vi "CalculateChargeDensity.vi"(6 "empty image":bool, 8 "Final":T2, 9 "Settings.LimitE":T1, 10 "MaxE":dbl, 11 "Z":dbl[][](graph)) -> (0 "Charge vs angle":cluster{"Ramp Pattern":dbl[], dbl[]}, 1 "Integrated spectrum (attoC/MeV or GeV?)":cluster{"Momentum [MeV/C]":dbl[], dbl[]}(graph), 2 "charge (sum)":dbl, 3 "charge density":dbl[][](array[numeric]), 5 "time: 2Dinter":u32)   [LabVIEW 2013]
uses:
  Controls/finalCalib--Cluster.ctl
  shared/OnOffTypeDef.ctl
  <vilib>/Analysis/8numeric.llb/1D Numeric Integration.vi
  <vilib>/gmath/interp.llb/Interpolate 2D (2d X,Y).vi
  <vilib>/Analysis/NI_AALPro.lvlib
  <vilib>/gmath/NI_Gmath.lvlib
panel:
  out "mask":dbl[][](graph)
  out "Out":dbl[][](array[numeric])
  out "xi":dbl[][](array[numeric])
  out "transposed array 2":dbl[][](graph)
  out "transposed array":dbl[][](graph)
  in  "error constant":errorcluster
  out "error":i32
  out "Intensity Graph":dbl[][](graph)
  out "time: spectra":u32
  out "charge (YSum)":dbl format="%0.4f"
  out "charge (spectra)":dbl format="%0.4f"
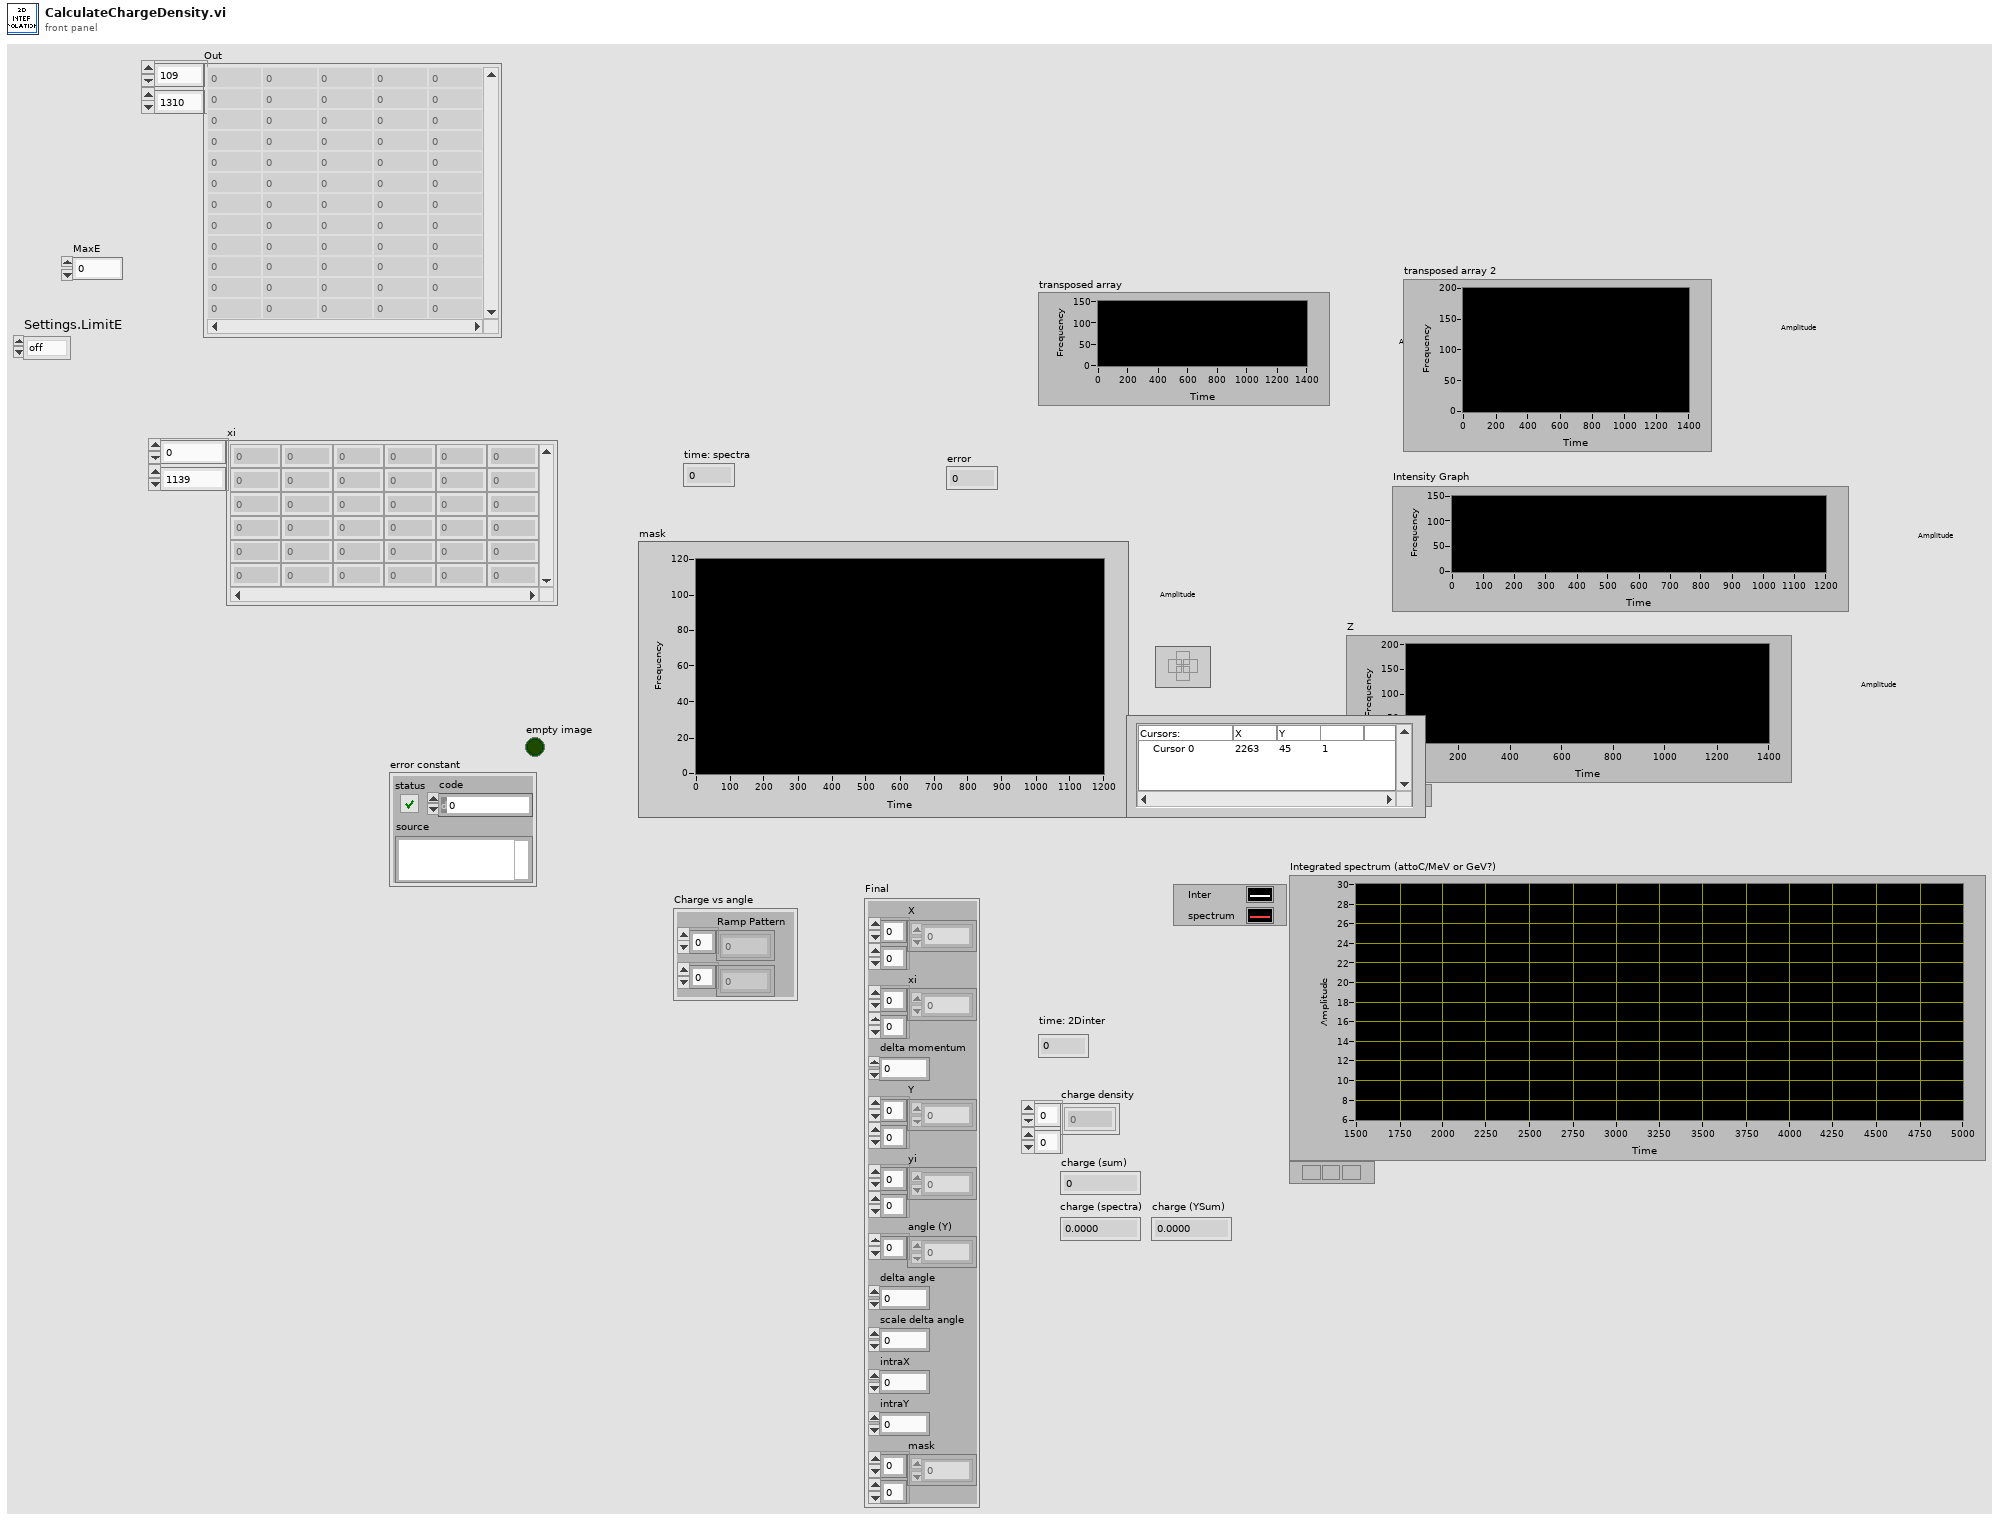
[diagram p1: front panel]
types:
  T1 = typedef "OnOffTypeDef.ctl" = enum16{"off", "on"}
  T2 = typedef "finalCalib--Cluster.ctl" = cluster{"X":dbl[][], "xi":dbl[][], "delta momentum":dbl, "Y":dbl[][], "yi":dbl[][], "angle (Y)":dbl[], "delta angle":dbl, "scale delta angle":dbl, "intraX":dbl, "intraY":dbl, "mask":dbl[][]}
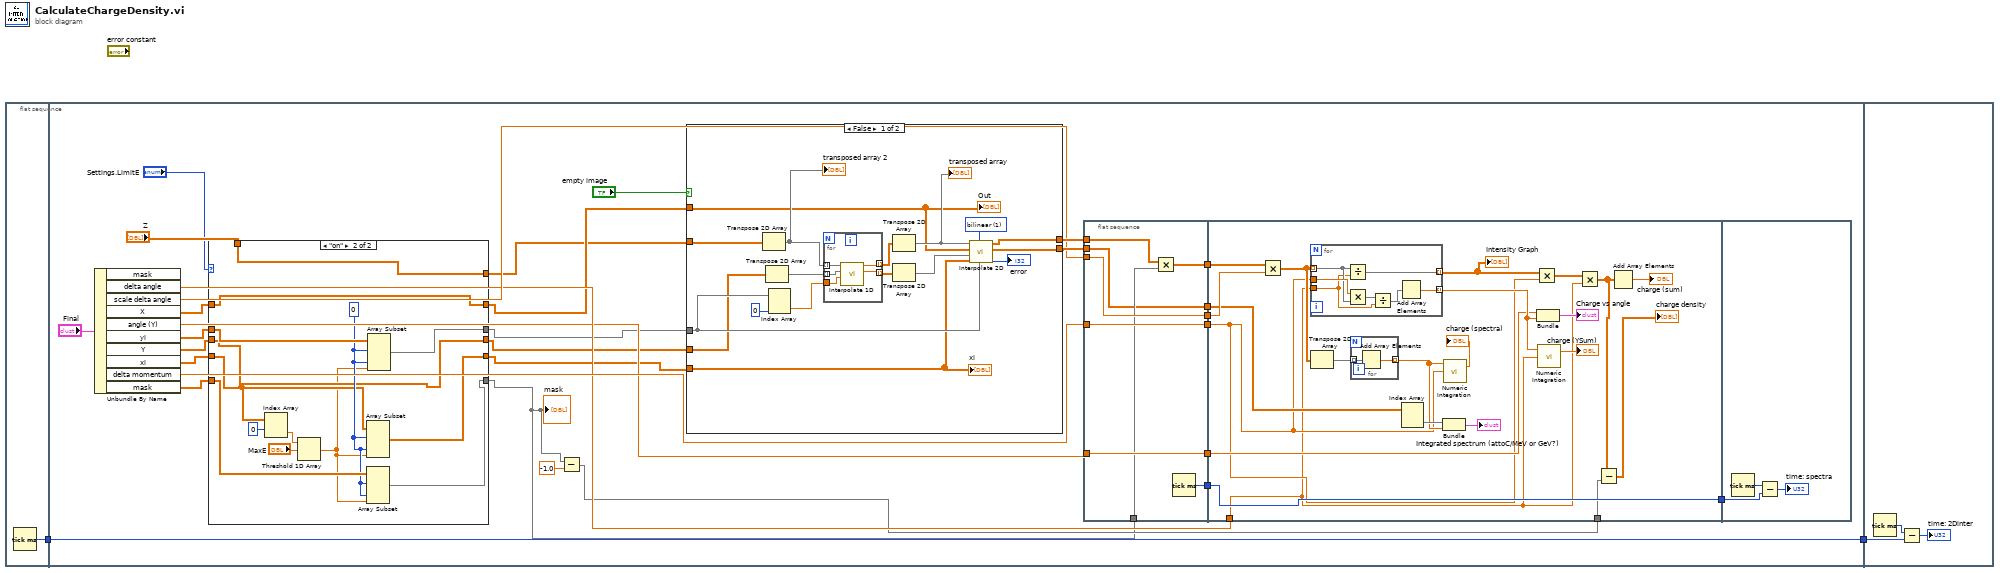
[diagram p0: block diagram]
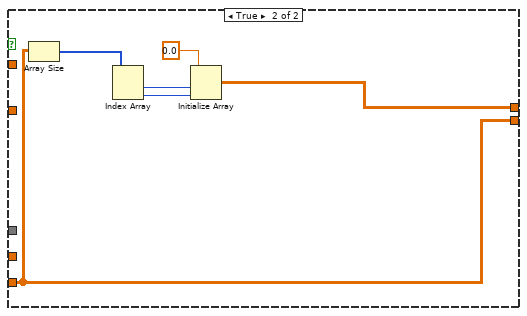
[diagram p3: hidden frame]
diagram:
  n1 = flat-sequence {
    tunnel: [w3] -> w2
    tunnel: w2 -> [w34]
    tunnel: [w34] -> w1
    tunnel: w1 -> [w126]
    frame #0 {
      n2 = Tick Count (ms)() -> (millisecond timer value=w3:u32)
    }
    frame #1 {
      n3 = Unbundle By Name("Final") -> ("delta angle"=w21:dbl, "scale delta angle"=w31:dbl, "X"=w16:dbl[][], "angle (Y)"=w20:dbl[], "yi"=w14:dbl[][], "Y"=w13:dbl[][], "xi"=w12:dbl[][], "delta momentum"=w23:dbl, "mask"=w8:dbl[][])  [unwired: 1 out]
      n4 = case shown="\"on\"" "Settings.LimitE" {
        tunnel: w16 -> [w40 w47]
        tunnel: [w40 w47] -> w15
        tunnel: w14 -> [w39 w54]
        tunnel: [w39 w53] -> w5
        tunnel: w13 -> [w38 w46]
        tunnel: [w38 w46] -> w6
        tunnel: w12 -> [w37 w45]
        tunnel: [w37 w52] -> w11
        tunnel: w8 -> [w36 w51]
        tunnel: [w36 w50] -> w7
        tunnel: "Z" -> [w35 w48]
        tunnel: [w35 w48] -> w9
        frame "off", Default {
        }
        frame "on" {
          w49 = 0 ("index")
          n5 = Index Array(array=w45, index (row)=0) -> (element=w43:dbl[])  [unwired: 1 in]
          n6 = Threshold 1D Array(2:"MaxE", 3:w43) -> (0:w41:dbl)  [unwired: 1 in]
          n7 = Array Subset(array=w45, index (row)=w49, index (col)=w49, length (col)=w41) -> (w52:dbl[][])  [unwired: 1 in]
          n8 = Array Subset(array=w51, index (row)=w49, index (col)=w49, length (col)=w41) -> (w50:dbl[][])  [unwired: 1 in]
          n9 = Array Subset(array=w54, index (row)=w49, index (col)=w49, length (col)=w41) -> (w53:dbl[][])  [unwired: 1 in]
        }
      }
      "mask" <- w7
      n10 = Subtract(x=w7, y=-1.0) -> (x-y=w17:dbl[][])
      n11 = case shown="False" "empty image" {
        tunnel: w15 -> [w56 _]
        tunnel: [w70 w81] -> w33
        tunnel: w11 -> [w57 w81]
        tunnel: w9 -> [w55 _]
        tunnel: [w71 w77] -> w32
        tunnel: w6 -> [w58 _]
        tunnel: w5 -> [w60 _]
        frame False {
          w66 = 1 items=["nearest", "bilinear", "bicubic", "bicubic spline"] ("method")
          n12 = Transpose 2D Array(2D array=w55) -> (transposed array=w59:dbl[][])
          "transposed array 2" <- w59
          n13 = Transpose 2D Array(2D array=w58) -> (transposed array=w68:dbl[][])
          n14 = Index Array(array=w60, index (col)=0 ("disabled index (col)")) -> (element=w67:dbl[])  [unwired: 1 in]
          n15 = for {
            tunnel: w59 -> [w76] mode=indexing
            tunnel: w68 -> [w75] mode=indexing
            tunnel: w67 -> [w74]
            tunnel: [w73] -> w64 mode=indexing
            tunnel: [w72] -> w63 mode=indexing
            n16 = call <vilib>:"Interpolate 1D.vi"("xi"=w74, "X"=w75, "Y"=w76) -> ("xi used"=w72:dbl[], "yi"=w73:dbl[])  [unwired: 6 in, 1 out]
          }
          n17 = Transpose 2D Array(2D array=w64) -> (transposed array=w62:dbl[][])
          "transposed array" <- w62
          n18 = Transpose 2D Array(2D array=w63) -> (transposed array=w61:dbl[][])
          n19 = call-poly <vilib>:"Interpolate 2D.vi"("yi"=w60, "method"=w66, "xi"=w57, "Y"=w61, "X"=w56, "Z"=w62) -> ("error"=→"error":i32, "xi used"=w70:dbl[][], "zi"=w71:dbl[][])  [unwired: 2 in, 1 out]
          "xi" <- w57
          "Out" <- w56
        }
        frame True {
          n20 = Array Size(array=w81) -> (size(s)=w80:i32[])
          n21 = Index Array(array=w80) -> (element #1=w79:i32, element #2=w78:i32)  [unwired: 2 in]
          n22 = Initialize Array(0.0 ("element"), w79, w78) -> (w77:dbl[][])
        }
      }
      n23 = flat-sequence {
        tunnel: w31 -> [w89]
        tunnel: w32 -> [w86]
        tunnel: w20 -> [w90]
        tunnel: w33 -> [w83]
        tunnel: [w83] -> w30
        tunnel: [w90] -> w29
        tunnel: [w84] -> w28
        tunnel: [w89] -> w27
        tunnel: [w88] -> w26
        tunnel: w23 -> [w87]
        tunnel: [w87] -> w22
        tunnel: w7 -> [w85]
        tunnel: w21 -> [w95]
        tunnel: w30 -> [w100]
        tunnel: w29 -> [w105]
        tunnel: w28 -> [w103]
        tunnel: w27 -> [w102]
        tunnel: w26 -> [w101]
        tunnel: [w101] -> w25
        tunnel: w22 -> [w97]
        tunnel: w17 -> [w92]
        tunnel: w25 -> [w123]
        frame #0 {
          n24 = Multiply(x=w86, y=w85) -> (x*y=w84:dbl[][])
          n25 = Tick Count (ms)() -> (millisecond timer value=w88:u32)
        }
        frame #1 {
          n26 = Multiply(x=w103, y=w102) -> (x*y=w99:dbl[][])
          n27 = for {
            tunnel: w99 -> [w117] mode=indexing
            tunnel: [w121] -> w106 mode=indexing
            tunnel: w97 -> [w118]
            tunnel: w95 -> [w116]
            tunnel: [w115] -> w98 mode=indexing
            n28 = Divide(x=w117, y=w116) -> (x/y=w115:dbl[])
            n29 = Multiply(x=w118, y=w117) -> (x*y=w120:dbl[])
            n30 = Divide(x=w120, y=w116) -> (x/y=w119:dbl[])
            n31 = Add Array Elements(numeric array=w119) -> (sum=w121:dbl)
          }
          "Intensity Graph" <- w98
          n32 = Transpose 2D Array(2D array=w99) -> (transposed array=w112:dbl[][])
          n33 = for {
            tunnel: w112 -> [w113] mode=indexing
            tunnel: [w114] -> w109 mode=indexing
            n34 = Add Array Elements(numeric array=w113) -> (sum=w114:dbl)
          }
          n35 = Index Array(array=w100) -> (element=w110:dbl[])  [unwired: 2 in]
          n36 = Bundle("xi"=w110, w109) -> (→"Integrated spectrum (attoC/MeV or GeV?)":cluster{"xi":dbl[], dbl[]})  [unwired: 1 in]
          n37 = call-poly <vilib>:"Numeric Integration.vi"("dt"=w97, "Input Array"=w109) -> ("result"=→"charge (spectra)":dbl)  [unwired: 1 in, 1 out]
          n38 = Multiply(x=w98, y=w97) -> (x*y=w96:dbl[][])
          n39 = Bundle("angle (Y)"=w105, w106) -> (→"Charge vs angle":cluster{"angle (Y)":dbl[], dbl[]})  [unwired: 1 in]
          n40 = call-poly <vilib>:"Numeric Integration.vi"("dt"=w95, "Input Array"=w106) -> ("result"=→"charge (YSum)":dbl)  [unwired: 1 in, 1 out]
          n41 = Multiply(x=w96, y=w95) -> (x*y=w93:dbl[][])
          n42 = Subtract(x=w93, y=w92) -> (x-y=→"charge density":dbl[][])
          n43 = Add Array Elements(numeric array=w93) -> (sum=→"charge (sum)":dbl)
        }
        frame #2 {
          n44 = Tick Count (ms)() -> (millisecond timer value=w124:u32)
          n45 = Subtract(x=w124, y=w123) -> (x-y=→"time: spectra":u32)
        }
      }
    }
    frame #2 {
      n46 = Tick Count (ms)() -> (millisecond timer value=w127:u32)
      n47 = Subtract(x=w127, y=w126) -> (x-y=→"time: 2Dinter":u32)
    }
  }
